vi "StagingSuperGUI.vi"() -> ()   [LabVIEW 2013]
uses:
  Device Driver/TRAServer/StatusTRA_TypDef.ctl
  shared programs/GUI_Template/GUI_master/tcp new data cluster.ctl
  Device Driver/TRAServer/TRAServer.lvclass
panel:
  in  "GUIdevice 13":string="StagingHallProbe"
  in  "Top Button":bool
  in  "Bottom Button":bool
  in  "GUIdevice 7":string="StagingHexapodPI"
  in  "GUIdevice 5":string="StagingLowPressure2"
  in  "GUIdevice 6":string="StagingTelescopePosition"
  in  "GUIdevice 22":string="StagingTelescopeImageLocation"
  in  "Position::22":dbl=47.0 caption="Telescope image location" min=-50.0 max=100.0
  in  "GUIdevice 20":string="StagingBeam2FocusLocation"
  in  "GUIdevice 19":string="StagingBeam1FocusLocation"
  in  "GUIdevice 18":string="StagingDelayStage"
  in  "Position::20":dbl=-0.0001 caption="Beam2Focus" min=-15.0 max=15.0 step=1.0 format="%#.6g"
  in  "Position::19":dbl=-0.0001 caption="Beam1Focus" min=0.0 max=100.0 step=1.0 format="%.6f"
  in  "position.Channel 1::18":dbl caption="DelayStage" min=0.0 max=50.0 step=0.01 format="%_6g"
  in  "EnergyOut::21":dbl caption="Energy Out" min=0.0 max=25.0 format="%.3p"
  in  "EnergyIn::21":dbl caption="Energy In" min=0.0 max=25.0 format="%.3p"
  in  "Position.Axis 2::17":dbl=-10.0 caption="M4stage"
  in  "Position.Axis 1::17":dbl=-10.0 caption="OAP1stage" min=-0.1 max=0.1
  in  "GUIdevice 17":string="StagingBeam1OAPMotors"
  in  "fire::15":string="fire2"
  in  "position.Channel 0::16":dbl=1.2974e-07 caption="Beam2 focus" min=0.0 max=0.0
  in  "GUIdevice 16":string="StagingOAP2Stage"
  in  "fire!!!":bool caption="fire"
  in  "GUIdevice 15":string="StagingShotControl"
  in  "Mode::15":bool caption="Mode"
  in  "stop 3":bool
  in  "stop 2":bool
  in  "stop":bool
  in  "Delay.ch ?":dbl=0.0005023 caption="Delay" format="%1.12f"
  in  "GUIdevice 14":string="StagingDG645_1"
  in  "Delay.ch e::14":dbl=0.0005023 caption="Delay" min=0.0 max=30.0 format="%1.12f"
  out "AI_mean.Channel 3::12":dbl=-0.02045096575 caption="voltage (DAQ)" min=0.0 max=30.0
  in  "relativemove.ypos::7":bool
  in  "relativemove.xpos::7":bool
  in  "relativemove.yneg::7":bool
  in  "relativemove.xneg::7":bool
  in  "relativemove.zpos::7":bool
  in  "relativemove.zneg::7":bool
  in  "relativemove.wpos::7":bool
  in  "relativemove.upos::7":bool
  in  "relativemove.uneg::7":bool
  in  "relativemove.vpos::7":bool
  in  "relativemove.vneg::7":bool
  in  "relativemove.wneg::7":bool
  out "Field::13":dbl=0.2555 caption="HallProbe"
  in  "takeData":bool
  out "AI_mean.Channel 0::12":dbl=-0.027788317856 caption="DAQ (V)"
  in  "GUIdevice 12":string="StagingDischargePower"
  in  "reprate::9":dbl=1.0 caption="reprate (Hz)"
  in  "Mode::9":enum16{"Continuous", "Single Shot"}(ring) caption="TriggerMode"
  in  "voltage.hv 2::11":dbl caption="voltage"
  in  "voltage.hv 1::11":dbl=-0.04046 caption="voltage"
  in  "GUIdevice 11":string="StagingDischargeHV"
  in  "trigger.message::10":string caption="Interlock Message"
  in  "installed.cap2::10":bool caption="CAP2"
  in  "installed.cap1::10":bool caption="CAP1"
  in  "GUIdevice 10":string="StagingInterlock"
  out "fire interlock::10":bool caption="Interlock"
  in  "enableLaser::9":bool caption="LaserTrigger"
  in  "GUIdevice 9":string="StagingShotControl"
  out "EnergyTransmission Chart":dbl(graph)=1.469369562583 caption="EnergyTransmission"
  in  "EnergyTransmission::21":dbl=1.469369562583 caption="Energy Transmission" min=0.0 max=0.0
  in  "GUIdevice 21":string="StagingAnalysis"
  out "originalZ::7":dbl=-0.7919 caption="originalZ" min=0.0 max=0.0
  out "originalY::7":dbl=3.9926 caption="originalY" min=0.0 max=0.0
  out "originalX::7":dbl=-10.0031 caption="originalX" min=0.0 max=0.0
  in  "wangle::7":dbl=-0.0001 caption="w" min=-5.0 max=5.0
  in  "vangle::7":dbl=0.0005 caption="v" min=-5.0 max=5.0
  in  "uangle::7":dbl caption="u" min=-5.0 max=5.0
  in  "stepsize::7":dbl=0.001 caption="stepsize" min=0.0 max=10.0
  in  "zpos::7":dbl=-0.794 caption="Z" min=-12.0 max=12.0
  in  "ypos::7":dbl=4.0 caption="Y" min=-20.0 max=20.0
  in  "device status::7":string="no scan" caption="Status"
  in  "xpos::7":dbl=-10.0 caption="X" min=-20.0 max=20.0
  in  "device status::6":string="no scan"
  in  "Position.Axis 1::6":dbl=47.0 caption="Telescope position" min=0.0 max=150.0
  out "valve::5":bool
  in  "pressure::5":dbl=117.14 caption="CAP2" min=0.0 max=200.0
  in  "discharge2::4":bool caption="CAP2"
  in  "discharge1::4":bool caption="CAP1"
  in  "device status::4":string="Initialized" caption="Discharge (NI Switch)"
  in  "GUIdevice 4":string="StagingNISwitch"
  out "Status.Axis 5::3":T1=enum."DISABLE" caption="Status"
  in  "Position.Axis 5::3":dbl=20.0 caption="compensation stage" min=-49.0 max=51.0
  in  "device status::3":string="Initialized"
  in  "GUIdevice 3":string="StagingTRA3"
  in  "pressure::2":dbl=0.06 caption="CAP1" min=0.0 max=200.0
  out "valve::2":bool caption="valve"
  out "pressureCap2::1":dbl=746.520248508741 caption="pressure Cap2" min=0.0 max=10.0
  out "pressureCap1::1":dbl=743.525107996803 caption="read (torr)" min=0.0 max=10.0
  in  "GUIdevice 2":string="StagingLowPressure1"
  in  "GUIdevice 1":string="StagingAnalysisSlow"
  in  "insert tag":bool=TRUE
  # "STAGING GRAPHICAL USER INTERFACE"
  # "Hexapod"
  # "Laser"
  # "Trigger"
  # "Magnet"
  # "Installed:"
  # "Pressure"
  # "SHOT CONTROL"
  # "set (torr)"
  # "Z"
  # "+"
  # "Y"
  # "+"
  # "-"
  # "+"
  # "-"
  # "-"
  # "X"
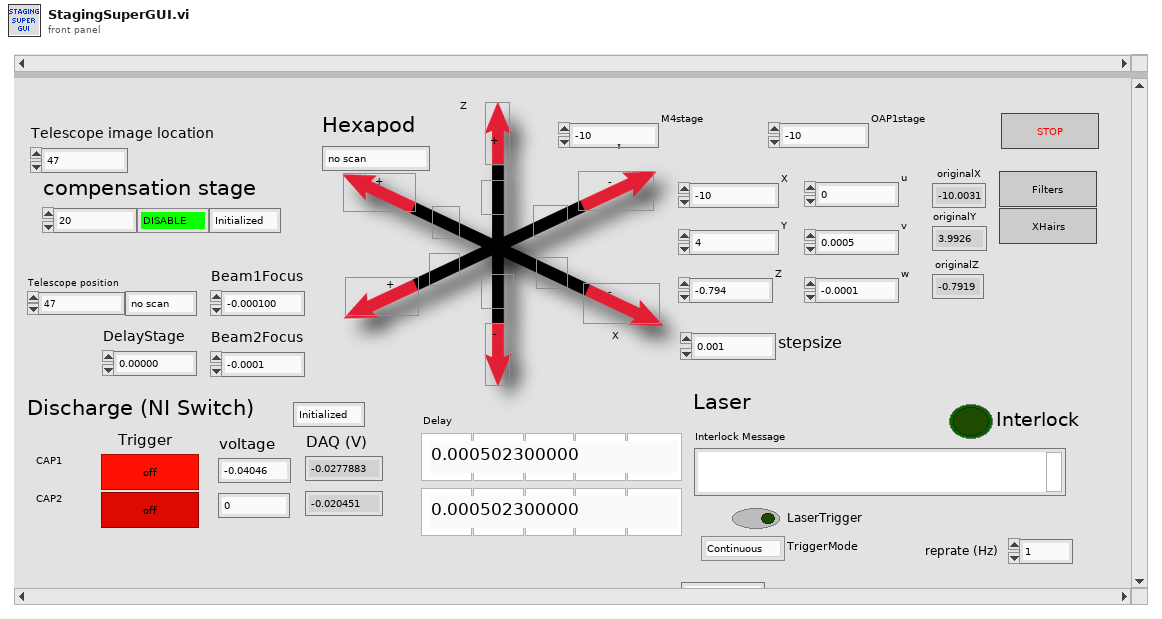
[diagram p1: front panel]
types:
  T1 = typedef "TRAServer.lvclass/StatusTRA_TypDef.ctl" = enum16{"NOT REFERENCED", "CONFIGURATION", "HOMING", "MOVING", "READY", "DISABLE", "JOGGING"}
  T2 = typedef "tcp new data cluster.ctl" = cluster{"EventEnum":enum16{"new data", "connection status update"}, "Device name":string}
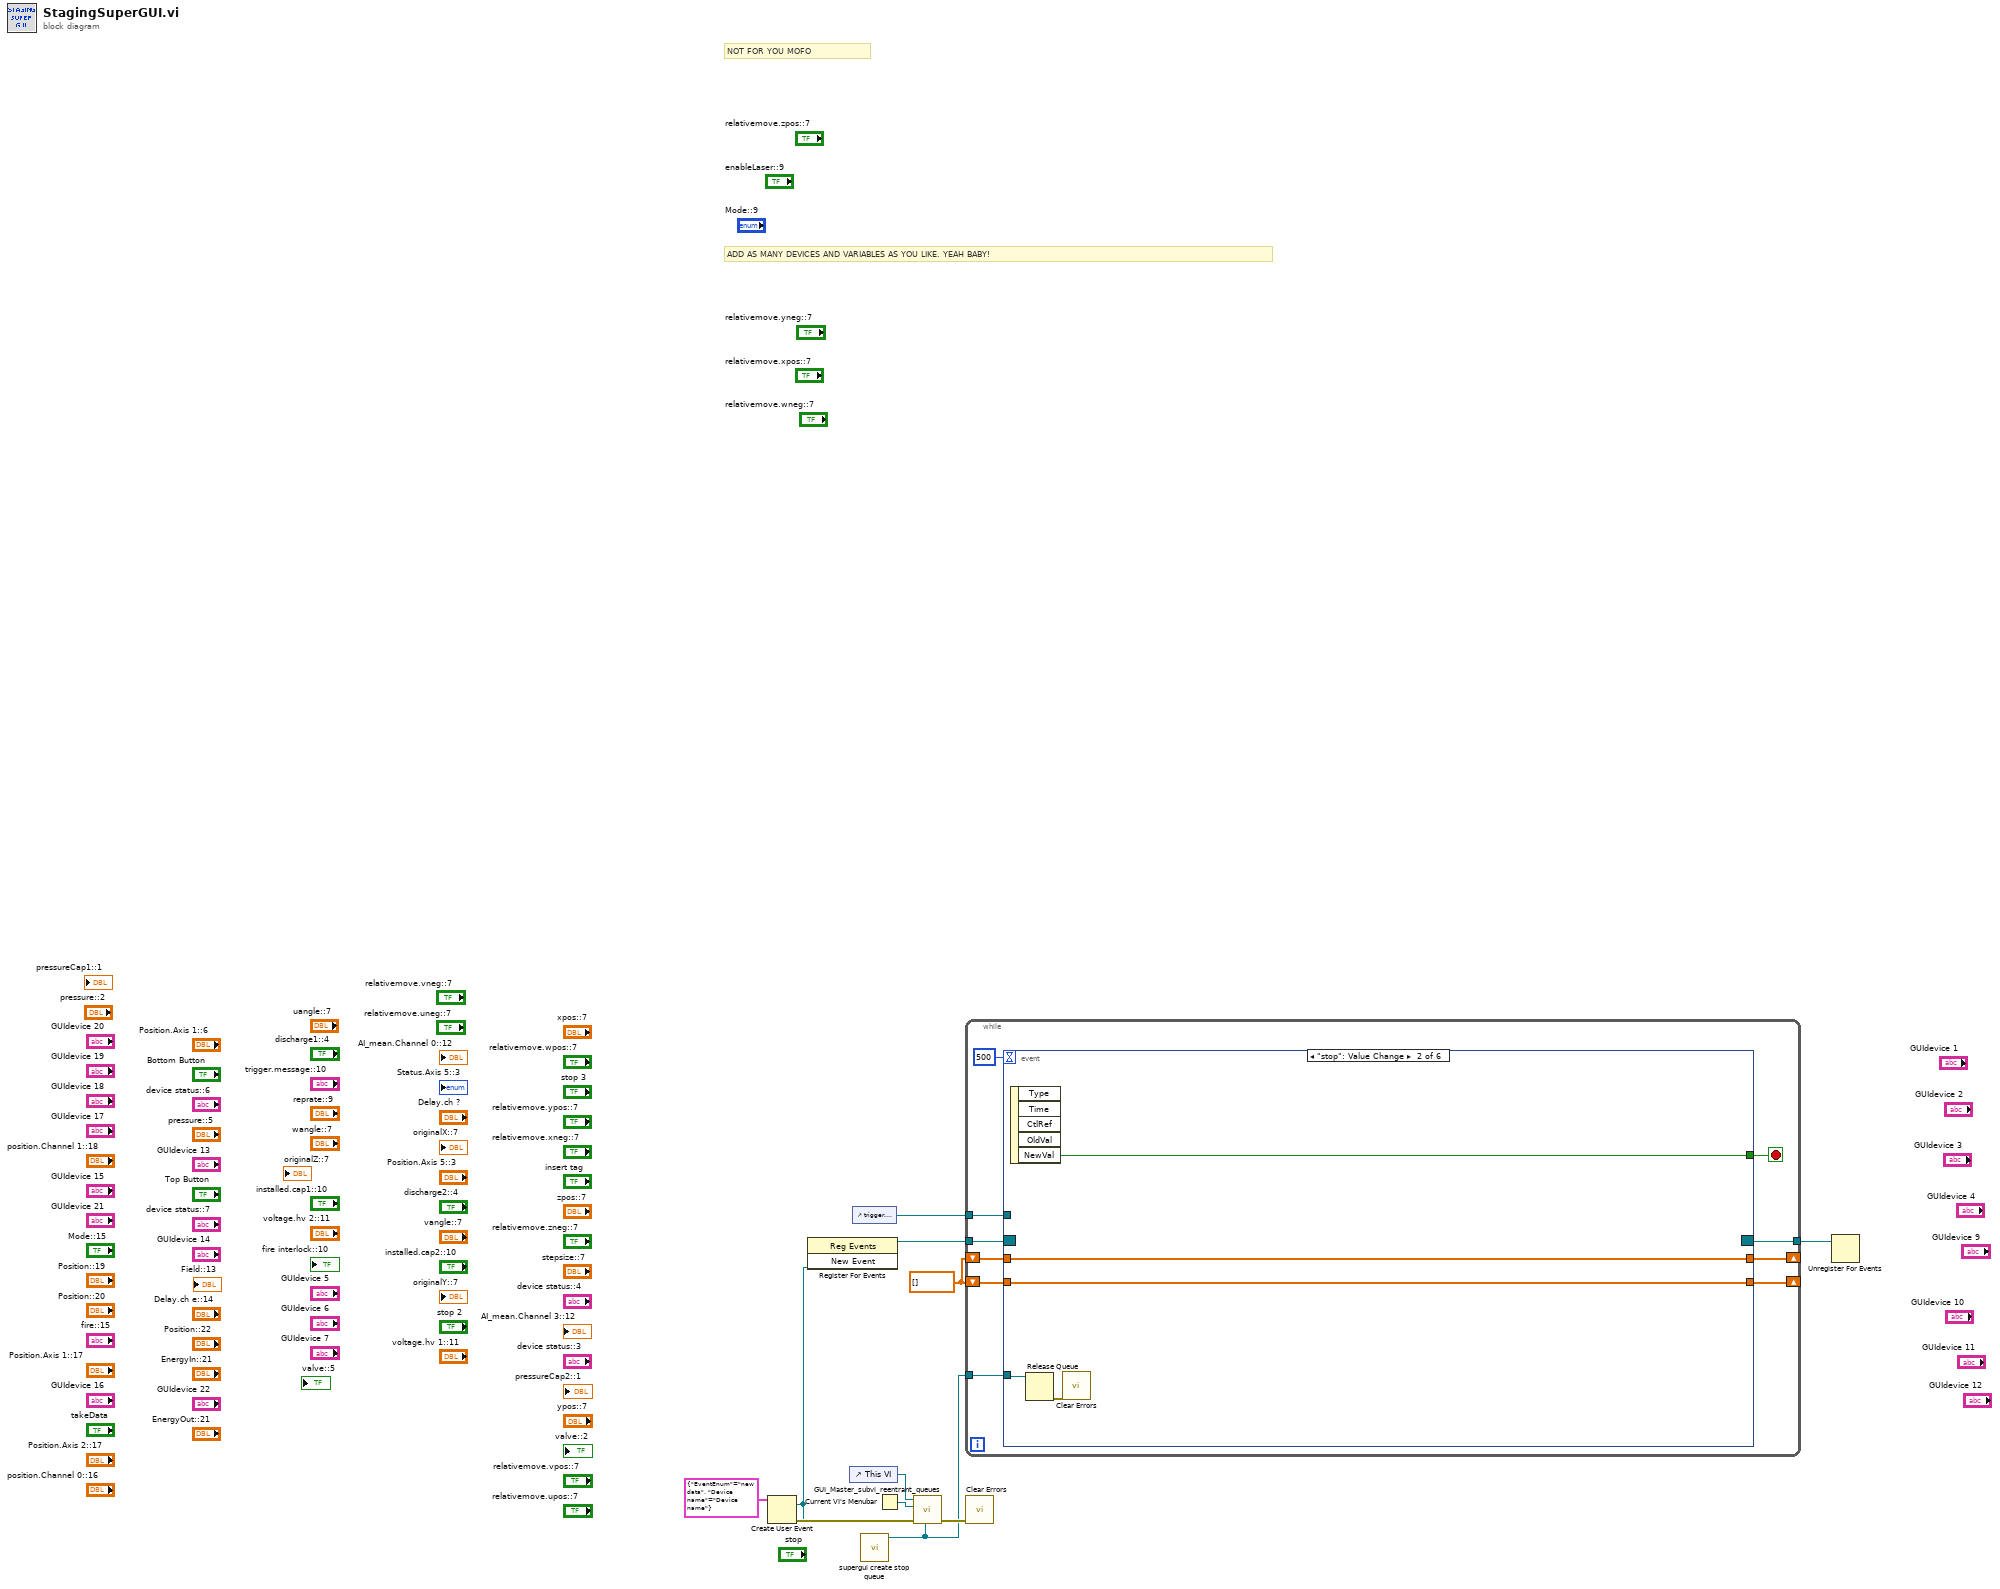
[diagram p0: block diagram]
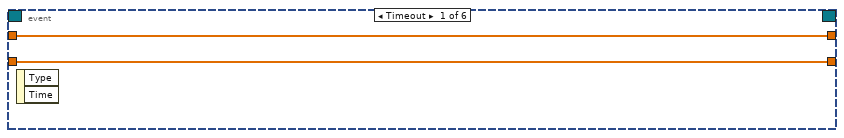
[diagram p2: hidden frame]
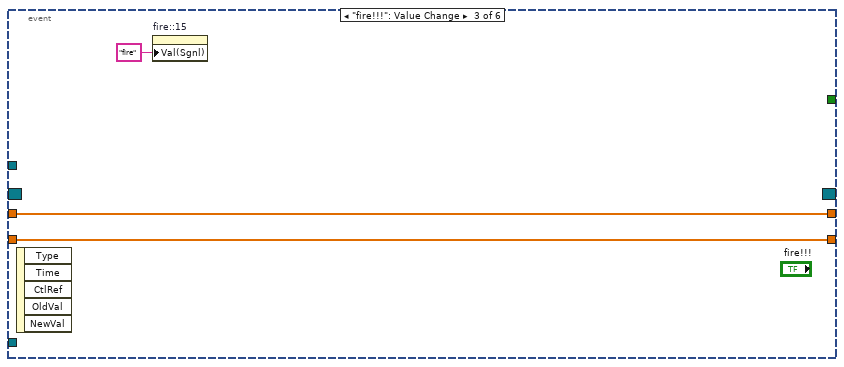
[diagram p3: hidden frame]
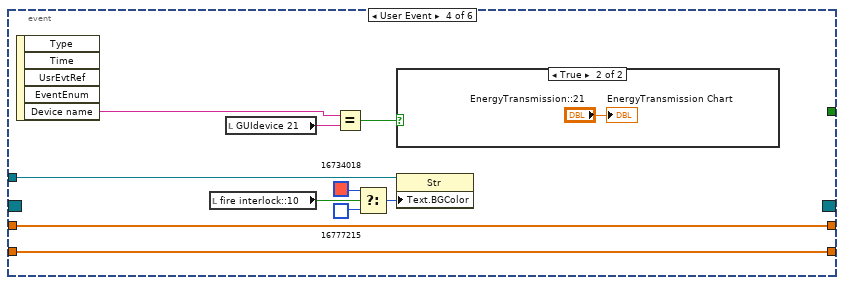
[diagram p4: hidden frame]
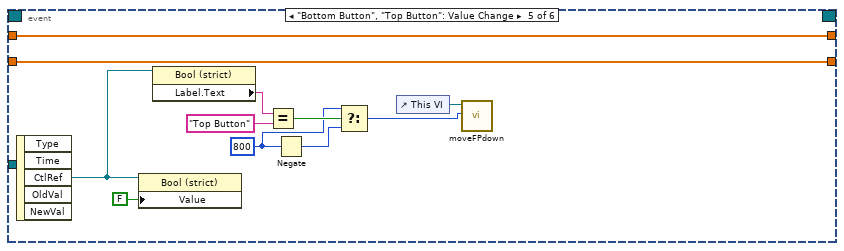
[diagram p6: hidden frame]
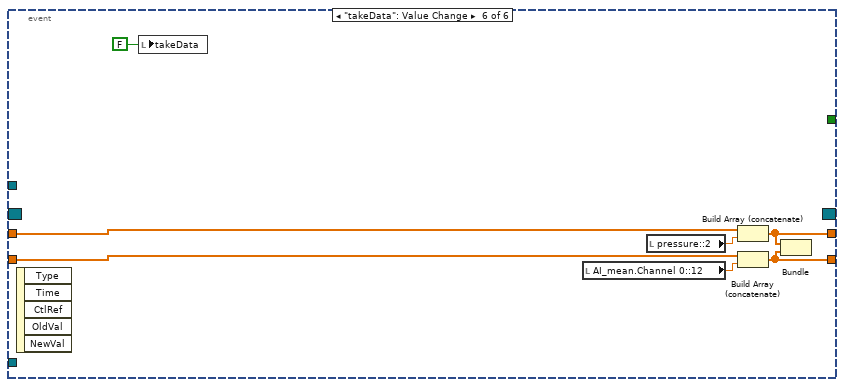
[diagram p7: hidden frame]
diagram:
  w6 = dbl[] []
  # "ADD AS MANY DEVICES AND VARIABLES AS YOU LIKE. YEAH BABY!"
  # "NOT FOR YOU MOFO"
  n1 = Create User Event(user event datatype=T2 {"EventEnum"=enum."new data", "Device name"="Device name"} ("New Event")) -> (user event=w3:refnum<user-event>, error out=w8:errorcluster)  [unwired: 1 in]
  n2 = register-events(w3) -> (reference out=w7:refnum<event-registration>)  [unwired: 2 in, 1 out]
  n3 = control-ref of="This VI"() -> (w11:refnum<vi>)
  n4 = control-ref of="trigger.message::10"() -> (w5:refnum<vi>)
  n5 = call "supergui create stop queue.vi"() -> ("STOP Queue out"=w1:refnum<queue>)  [unwired: 11 in]
  n6 = Current VI's Menubar() -> (w10:refnum<k9>)
  n7 = call "GUI_Master_subvi_reentrant_queues.vi"("STOP Queue in"=w1, "error in (no error)"=w8, "tcp data event"=w3, "Caller menu reference"=w10, "Caller VI ref"=w11) -> ("error out"=w2:errorcluster)  [unwired: 6 in]
  n8 = while {
    tunnel: w7 -> [w21]
    shift-right: [w19] -> _
    shift-left: w6 -> [w18]
    shift-right: [w17] -> _
    shift-left: w6 -> [w16]
    tunnel: w5 -> [w15]
    tunnel: [w14] -> w4
    tunnel: w1 -> [w12]
    stop <- w20 stop-if-true
    n9 = event shown="[1] \"stop\": Value Change" {
      selector: w21 -> [_ _ _ _ _ _]
      dyn-events: [_ _ _ _ _ _] -> w14
      timeout: 500 -> [_ _ _ _ _ _]
      tunnel: [_ w28 _ _ _ _] -> w20
      tunnel: [w23 w26 w30 w37 w43 w56] -> w19
      tunnel: w18 -> [w23 w26 w30 w37 w43 w60]
      tunnel: [w22 w27 w31 w38 w44 w57] -> w17
      tunnel: w16 -> [w22 w27 w31 w38 w44 w58]
      tunnel: w15 -> [_ _ _ w36 _ _]
      tunnel: w12 -> [_ w25 _ _ _ _]
      event Timeout {
        n10 = event-data() -> ()  [unwired: 1 in, 2 out]
      }
      event "stop": Value Change {
        n11 = event-data() -> ("NewVal"=w28:bool)  [unwired: 1 in, 4 out]
        n12 = Release Queue(queue=w25) -> (error out=w24:errorcluster)  [unwired: 2 in, 2 out]
        n13 = call <vilib>:"Clear Errors.vi"("error in (no error)"=w24) -> ()  [unwired: 6 in, 1 out]
      }
      event "fire!!!": Value Change {
        n14 = event-data() -> ()  [unwired: 1 in, 5 out]
        n15 = property on="fire::15" class="Str"("Val(Sgnl)"="fire" ("Value (Signaling)")) -> ()  [unwired: 2 in, 2 out]
      }
      event User Event {
        n16 = event-data() -> ("Device name"=w41:string)  [unwired: 1 in, 4 out]
        n17 = local read "fire interlock::10"() -> (w32:bool)
        n18 = local read "GUIdevice 21"() -> (w40:string)
        n19 = Equal?(x=w41, y=w40) -> (x = y?=w39:bool)
        n20 = Select(t=u32 16734018, s=w32, f=u32 16777215) -> (s? t:f=w33:u32)
        n21 = case shown="True" w39 {
          frame False {
          }
          frame True {
            "EnergyTransmission Chart" <- "EnergyTransmission::21"
          }
        }
        n22 = property class="Str"(reference=w36, "Text.BGColor"=w33) -> ()  [unwired: 1 in, 2 out]
      }
      event "Bottom Button", "Top Button": Value Change {
        w47 = i16 800 ("y")
        n23 = event-data() -> ("CtlRef"=w51:refnum<vi>)  [unwired: 1 in, 4 out]
        n24 = property class="Bool (strict)"(reference=w51, "Value"=FALSE) -> ()  [unwired: 1 in, 2 out]
        n25 = property class="Bool (strict)"(reference=w51) -> ("Label.Text"=w50:string)  [unwired: 1 in, 2 out]
        n26 = Equal?(x=w50, y="Top Button") -> (x = y?=w48:bool)
        n27 = Negate(x=w47) -> (-x=w46:i16)
        n28 = Select(t=w47, s=w48, f=w46) -> (s? t:f=w45:i16)
        n29 = control-ref of="This VI"() -> (w53:refnum<vi>)
        n30 = call "moveFPdown.vi"("y"=w45, "This VI"=w53) -> ()  [unwired: 9 in, 1 out]
      }
      event "takeData": Value Change {
        n31 = event-data() -> ()  [unwired: 1 in, 5 out]
        n32 = local write "takeData"(FALSE ("takeData")) -> ()
        n33 = local read "AI_mean.Channel 0::12"() -> (w54:dbl)
        n34 = local read "pressure::2"() -> (w59:dbl)
        n35 = Build Array (concatenate)(w58, w59) -> (w57:dbl[])
        n36 = Build Array (concatenate)(w60, w54) -> (w56:dbl[])
        n37 = Bundle(w57, w56) -> ()  [unwired: 1 in, 1 out]
      }
    }
  }
  n38 = call <vilib>:"Clear Errors.vi"("error in (no error)"=w2) -> ()  [unwired: 6 in, 1 out]
  n39 = Unregister For Events(event registration refnum=w4) -> ()  [unwired: 1 in, 1 out]
